vi "VMI_set_delay_list.vi"(5 "Table":string[][](table), 6 "Pump":dbl, 7 "Probe":dbl) -> (0 "Number delays":i32, 1 "Delay_list":dbl[][](array[numeric]), 2 "Delay_full_dir":string[](array[string]), 3 "First Point":dbl, 4 "Delay_dir_list":string[](array[string]))   [LabVIEW 2018]
panel:
  out "size(s)":i32[](array[numeric])
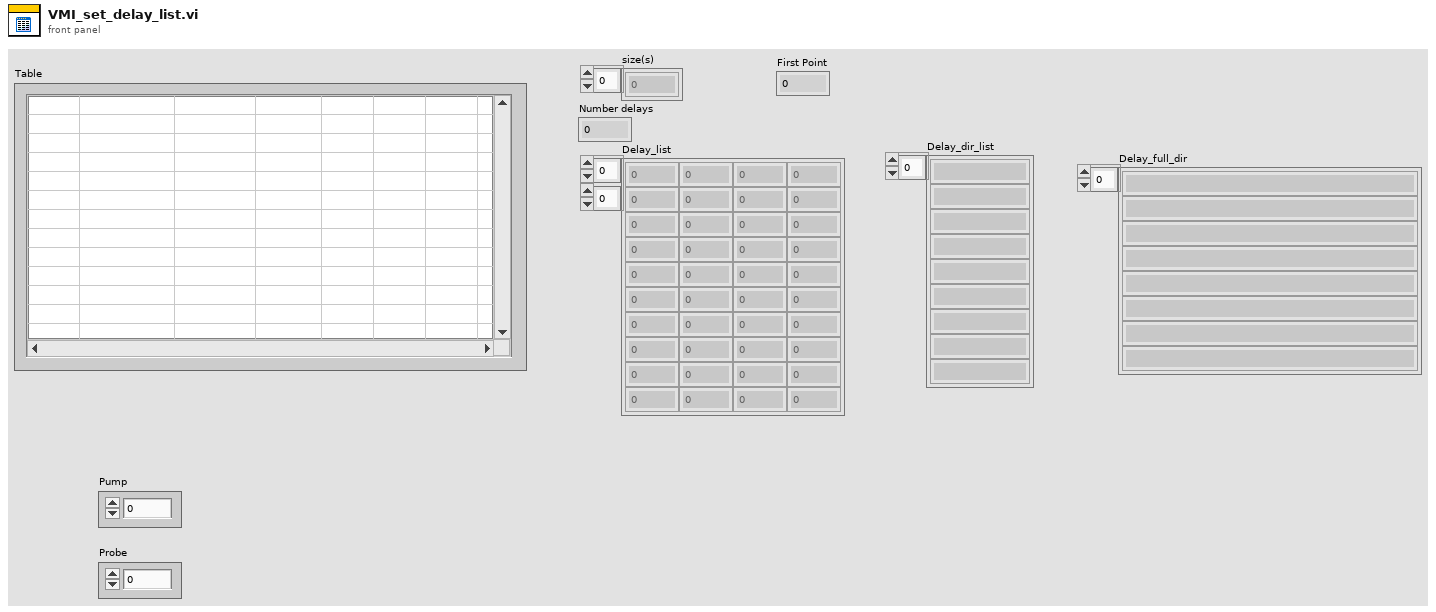
[diagram p1: front panel]
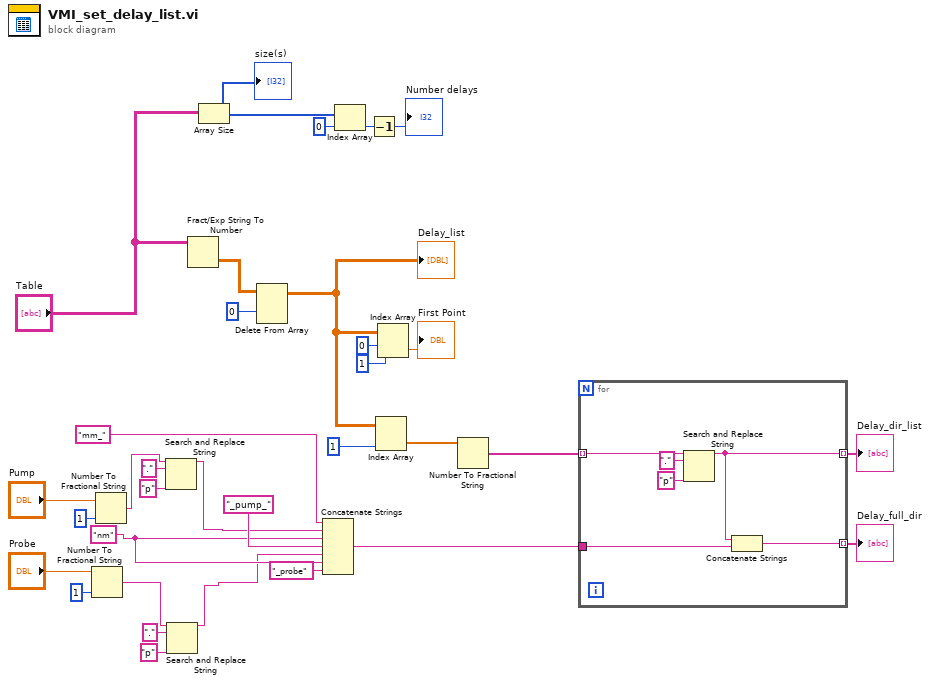
[diagram p0: block diagram]
diagram:
  w12 = "nm" ("string")
  n1 = Number To Fractional String(number="Probe", precision (6)=i16 1) -> (F-format string=w2:string)  [unwired: 2 in]
  n2 = Number To Fractional String(number="Pump", precision (6)=i16 1) -> (F-format string=w6:string)  [unwired: 2 in]
  n3 = Search and Replace String(input string=w6, search string=".", replace string="p" ("replace string (\"\")")) -> (result string=w5:string)  [unwired: 5 in, 3 out]
  n4 = Search and Replace String(input string=w2, search string=".", replace string="p" ("replace string (\"\")")) -> (result string=w1:string)  [unwired: 5 in, 3 out]
  n5 = Fract/Exp String To Number(string="Table") -> (number=w25:dbl[][])  [unwired: 3 in, 1 out]
  n6 = Array Size(array="Table") -> (size(s)=w33:i32[])
  "size(s)" <- w33
  n7 = Delete From Array(array=w25, index (row)=0) -> (array with subset deleted=w23:dbl[][])  [unwired: 2 in, 1 out]
  "Delay_list" <- w23
  n8 = Concatenate Strings("mm_", w5, w12, "_pump_" ("string"), w1, w12, "_probe" ("string")) -> (w10:string)
  n9 = Index Array(array=w33, index=0) -> (element=w31:i32)
  n10 = Decrement(x=w31) -> (x-1=→"Number delays":i32)
  n11 = Index Array(array=w23, index (col)=1 ("index (row)")) -> (element=w21:dbl[])  [unwired: 1 in]
  n12 = Index Array(array=w23, index (row)=0, index (col)=1 ("disabled index (col)")) -> (element=→"First Point":dbl)
  n13 = Number To Fractional String(number=w21) -> (F-format string=w20:string[])  [unwired: 3 in]
  n14 = for {
    tunnel: w20 -> [w39] mode=indexing
    tunnel: [w35] -> w19 mode=indexing
    tunnel: w10 -> [w36]
    tunnel: [w34] -> w9 mode=indexing
    n15 = Search and Replace String(input string=w39, search string=".", replace string="p" ("replace string (\"\")")) -> (result string=w35:string)  [unwired: 5 in, 3 out]
    n16 = Concatenate Strings(w35, w36) -> (w34:string)
  }
  "Delay_dir_list" <- w19
  "Delay_full_dir" <- w9
